vi "LVIS_ErrorMsg.vi"(8 "Error In":errorcluster, 9 "Response":string, 10 "Send CRC":string, 11 "Success?":bool) -> (0 "Error out":errorcluster)   [LabVIEW 2015]
doc: "If the send process was not successful, checks for the culprit and throws an appropiate error."
uses:
  Globals/LVIS_DcGlobals.vi
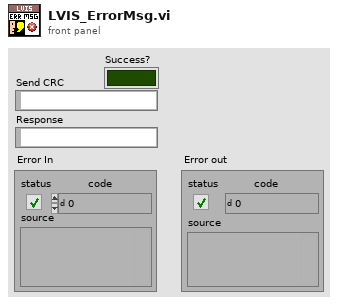
[diagram p1: front panel]
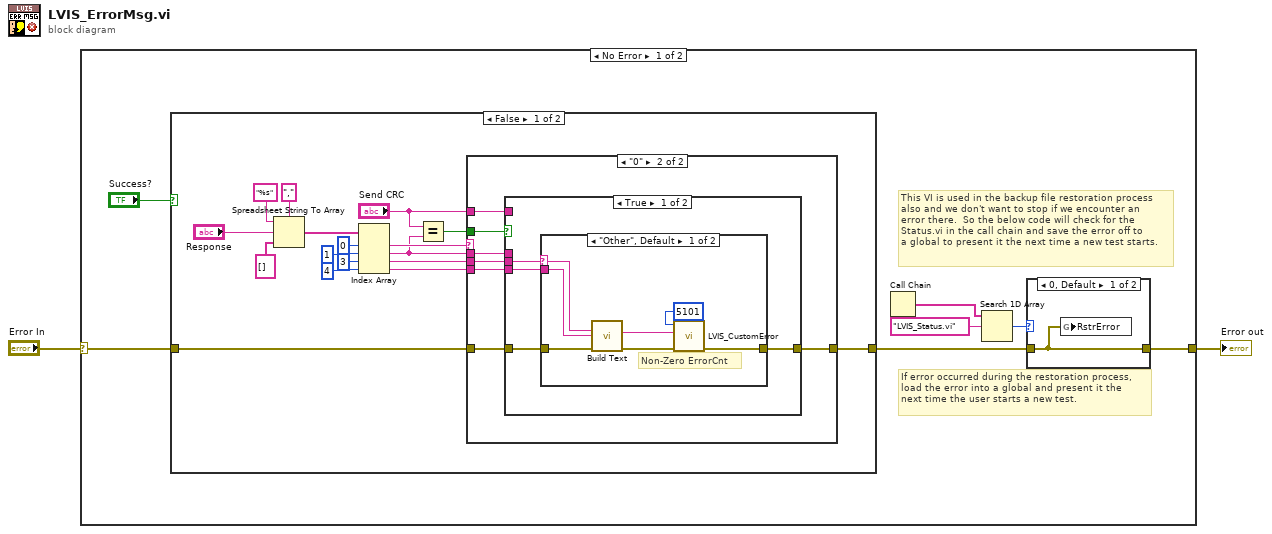
[diagram p0: block diagram]
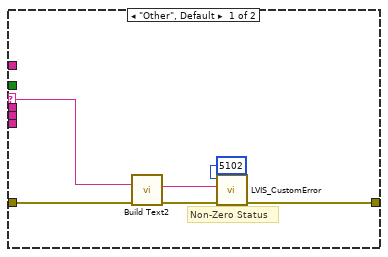
[diagram p3: hidden frame]
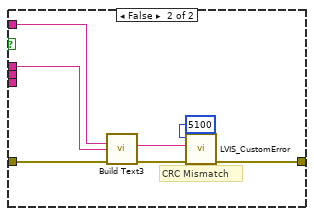
[diagram p5: hidden frame]
diagram:
  n1 = case shown="No Error" "Error In" {
    selector: "Error In" -> [w9 w62]
    tunnel: [w4 w62] -> w2
    frame No Error {
      # "This VI is used in the backup file restoration process\nalso and we don't want to stop if we encounter an\nerror there.  So the below code will check for the \nStatus.vi in the call chain and save the error off to\na global to present it the next time a new test starts."
      # "If error occurred during the restoration process,\nload the error into a global and present it the\nnext time the user starts a new test."
      n2 = case shown="False" "Success?" {
        tunnel: w9 -> [w28 w61]
        tunnel: [w27 w61] -> w5
        frame False {
          n3 = Spreadsheet String To Array(delimiter (Tab)=",", format string="%s", spreadsheet string="Response", array type (2D Dbl)=string[] []) -> (array=w23:string[])
          n4 = Index Array(array=w23, index #1=0 ("index"), index #2=1 ("index"), index #3=3 ("index"), index #4=4 ("index")) -> (element #1=w17:string, element #2=w15:string, element #3=w12:string, element #4=w13:string)
          n5 = Equal?(x="Send CRC", y=w15) -> (x = y?=w16:bool)
          n6 = case shown="\"0\"" w17 {
            selector: w17 -> [w29 _]
            tunnel: w28 -> [w32 w41]
            tunnel: [w33 w40] -> w27
            tunnel: w16 -> [_ w39]
            tunnel: w15 -> [_ w38]
            tunnel: "Send CRC" -> [_ w37]
            tunnel: w12 -> [_ w36]
            tunnel: w13 -> [_ w35]
            frame "Other", Default {
              # "Non-Zero Status"
              n7 = call "Build Text2"("Status"=w29, "error in (no error)"=w32) -> ("Result"=w30:string, "error out"=w31:errorcluster)  [unwired: 12 in]
              n8 = call "LVIS_CustomError.vi"("error in (no error)"=w31, "Addiitional Info"=w30, "Code"=5102) -> ("error out"=w33:errorcluster)  [unwired: 8 in]
            }
            frame "0" {
              n9 = case shown="True" w39 {
                tunnel: w41 -> [w45 w57]
                tunnel: [w42 w56] -> w40
                tunnel: w38 -> [_ w55]
                tunnel: w37 -> [_ w54]
                tunnel: w36 -> [w43 _]
                tunnel: w35 -> [w44 _]
                frame True {
                  n10 = case shown="\"Other\", Default" w43 {
                    selector: w43 -> [w46 _]
                    tunnel: w45 -> [w49 w53]
                    tunnel: w44 -> [w47 _]
                    tunnel: [w48 w53] -> w42
                    frame "Other", Default {
                      # "Non-Zero ErrorCnt"
                      n11 = call "Build Text"("Count"=w46, "Msg"=w47, "error in (no error)"=w49) -> ("Result"=w50:string, "error out"=w51:errorcluster)  [unwired: 11 in]
                      n12 = call "LVIS_CustomError.vi"("error in (no error)"=w51, "Addiitional Info"=w50, "Code"=5101) -> ("error out"=w48:errorcluster)  [unwired: 8 in]
                    }
                    frame "0" {
                    }
                  }
                }
                frame False {
                  # "CRC Mismatch"
                  n13 = call "Build Text3"("Sent"=w54, "Received"=w55, "error in (no error)"=w57) -> ("Result"=w58:string, "error out"=w59:errorcluster)  [unwired: 11 in]
                  n14 = call "LVIS_CustomError.vi"("error in (no error)"=w59, "Addiitional Info"=w58, "Code"=5100) -> ("error out"=w56:errorcluster)  [unwired: 8 in]
                }
              }
            }
          }
        }
        frame True {
        }
      }
      n15 = Call Chain() -> (call chain=w6:string[])
      n16 = Search 1D Array(1D array=w6, element="LVIS_Status.vi") -> (index of element=w3:i32)  [unwired: 1 in]
      n17 = case shown="0, Default" w3 {
        tunnel: w5 -> [w10 w11]
        tunnel: [w10 w11] -> w4
        frame 0, Default {
          n18 = global write "LVIS_DcGlobals.vi" "RstrError"(w10) -> ()
        }
        frame -1 {
        }
      }
    }
    frame Error {
    }
  }
  "Error out" <- w2
